vi "iBs.vi"(0 "Laser On/Off":bool=TRUE, 1 "VISA resource name":refnum<visa-resource-name>="COM4") -> ()   [LabVIEW 2016]
uses:
  <vilib>/Instr/_visa.llb/VISA Configure Serial Port (Instr).vi
panel:
  in  "Laser On/Off 2":bool=TRUE
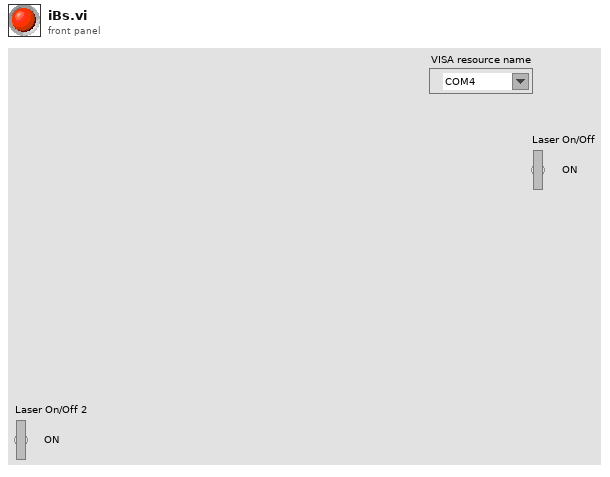
[diagram p1: front panel]
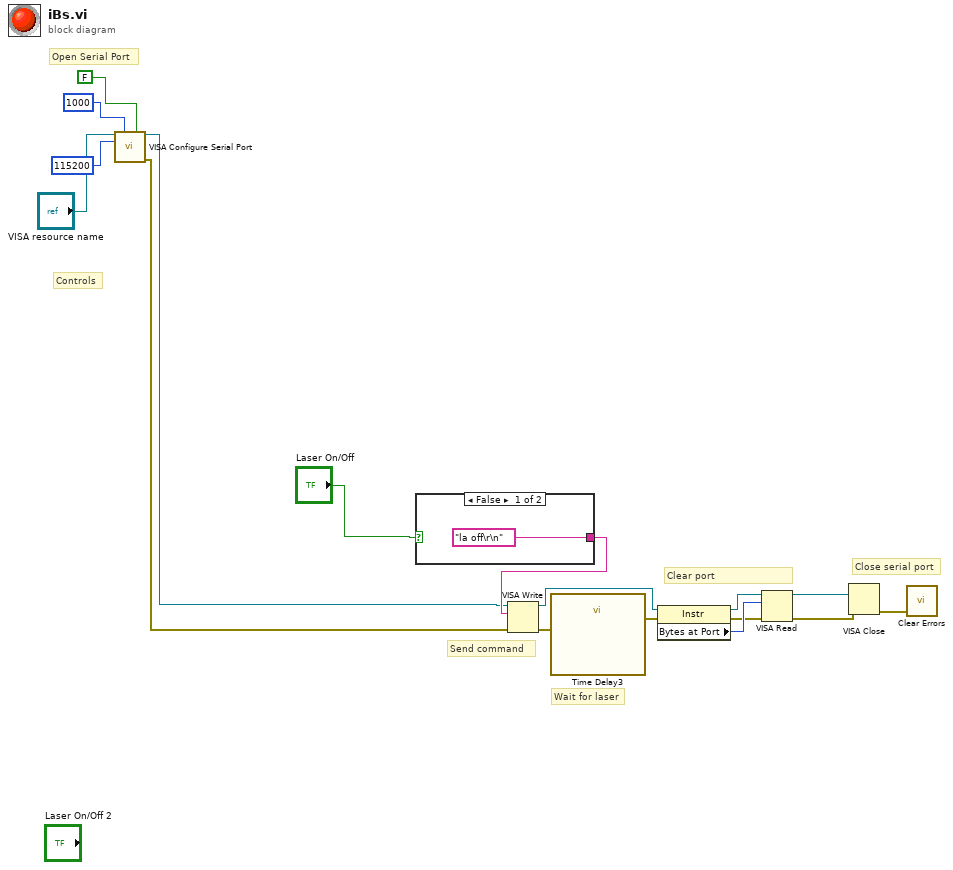
[diagram p0: block diagram]
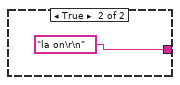
[diagram p2: hidden frame]
diagram:
  # "Close serial port"
  # "Clear port"
  # "Wait for laser"
  # "Send command"
  # "Controls"
  # "Open Serial Port"
  n1 = call-poly "VISA Configure Serial Port"("VISA resource name"="VISA resource name", "timeout (10sec)"=u32 1000, "Enable Termination\nChar (T)"=FALSE ("Enable Termination\nChar (T)"), "baud rate (9600)"=u32 115200) -> ("VISA resource name out"=w6:refnum<visa-resource-name>, "error out"=w5:errorcluster)  [unwired: 10 in]
  n2 = case shown="False" "Laser On/Off" {
    tunnel: ["la off\r\n" "la on\r\n"] -> w7
    frame False {
    }
    frame True {
    }
  }
  n3 = VISA Write(VISA resource name=w6, write buffer=w7, error in (no error)=w5) -> (VISA resource name out=w8:refnum<visa-resource-name>, error out=w10:errorcluster)  [unwired: 1 out]
  n4 = call "Time Delay3"("error in (no error)"=w10) -> ("error out"=w9:errorcluster)  [unwired: 10 in]
  n5 = property class="Instr"(reference=w8, error in=w9) -> (reference out=w13:refnum<visa-resource-name>, error out=w11:errorcluster, "Bytes at Port"=w12:u32)
  n6 = VISA Read(VISA resource name=w13, byte count=w12, error in (no error)=w11) -> (VISA resource name out=w4:refnum<visa-resource-name>, error out=w3:errorcluster)  [unwired: 2 out]
  n7 = VISA Close(VISA resource name=w4, error in (no error)=w3) -> (error out=w1:errorcluster)
  n8 = call <vilib>:"Clear Errors.vi"("error in (no error)"=w1) -> ()  [unwired: 5 in, 2 out]
